vi "Keithley 648X Series Alternating Voltage Resistance Test.vi"() -> ()   [LabVIEW 2021]
doc: "This example shows how to configure a measurement, set up triggering, trigger a measurement, and retrieve a measurement. It shows how to use the low-level Data VIs to retrieve data from the instrument.\n\n<b>Note:</b>\nThis VI is only valid for Keithley 6487."
uses:
  <instrlib>/Keithley 648X Series/Keithley 648X Series.lvlib
panel:
  in  "Upper Measurement Range":u16(ring) items=["20mA", "2mA", "200uA", "20uA", "2uA", "200nA", "20nA", "2nA"]
  out "AV Measurement Results":cluster{dbl[], dbl[]}(graph)
  out "AV Amplitude Results":dbl[](array[numeric])
  in  "Enable Zero Check":bool
  in  "Measurement Time":dbl=6.0
  in  "Enable One Shot Mode":bool
  in  "AV Units":u16(ring)=1 items=["Amps", "Ohms"]
  in  "AV Measurement Cycles":i32=5
  in  "AV Pulse Time":dbl=10.0
  in  "AV High Voltage":dbl=5.0
  in  "Serial Configuration":T1={"Baud Rate"=9600, "Parity"=0, "Data Bits"=8, "Stop Bits"=10, "Flow Control"=0} {"Flow Control" items=["None", "XON/XOFF", "RTS/CTS", "XON/XOFF & RTS/CTS", "DTR/DSR", "XON/XOFF & DTR/DSR"]; "Stop Bits" items=["1.0"=10, "1.5"=15, "2.0"=20]; "Data Bits" items=["7"=7, "8"=8]; "Parity" items=["None", "Odd", "Even", "Mark", "Space"]; "Baud Rate" items=["300"=300, "600"=600, "1200"=1200, "2400"=2400, "4800"=4800, "9600"=9600, "19200"=19200]}
  in  "VISA resource name":refnum<visa-resource-name>
  # "(c) 2017 National Instruments.  ALL RIGHTS RESERVED."
  # "Measurement time is restricted\nto  0.02, 0.1, 1, 6, and 60 PLC\nduring A-V ohms mode."
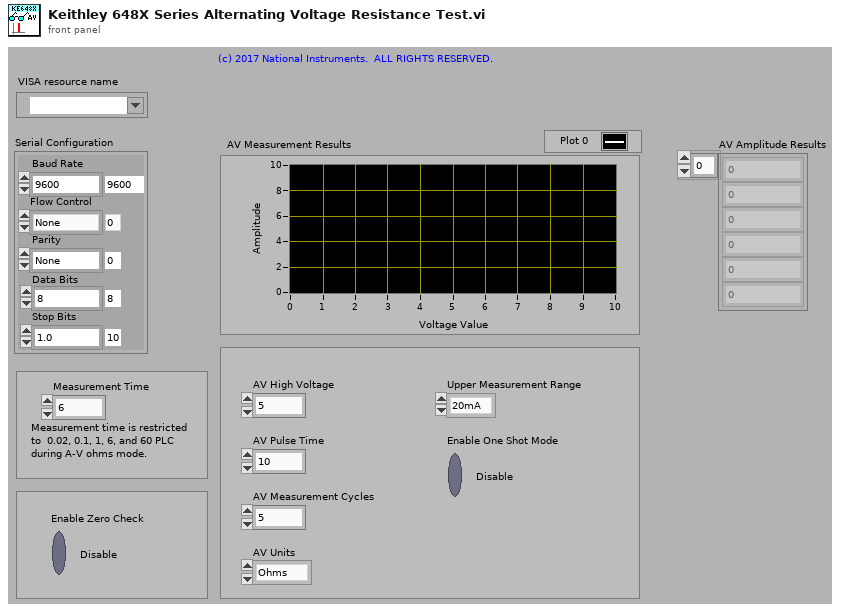
[diagram p1: front panel]
types:
  T1 = cluster{"Baud Rate":u32, "Parity":u16, "Data Bits":u16, "Stop Bits":u16, "Flow Control":u16}
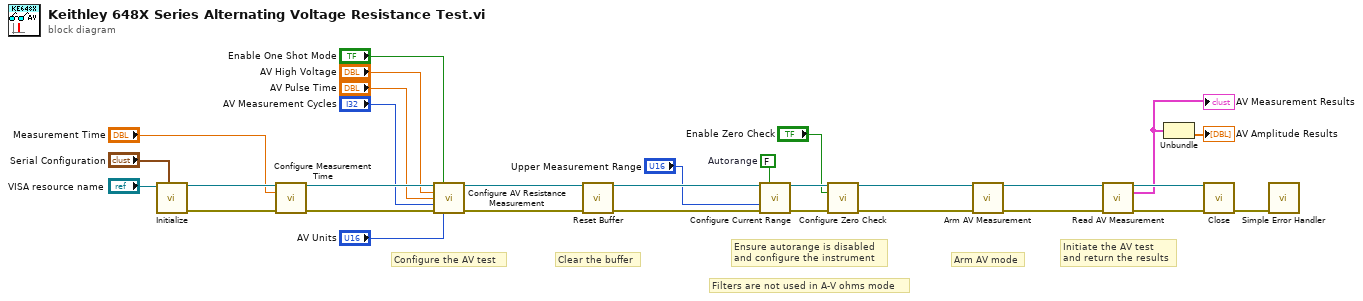
[diagram p0: block diagram]
diagram:
  w23 = FALSE  # Autorange
  # "Clear the buffer"
  # "Configure the AV test"
  # "Initiate the AV test\nand return the results"
  # "Arm AV mode"
  # "Ensure autorange is disabled\nand configure the instrument"
  # "Filters are not used in A-V ohms mode"
  n1 = call <instrlib>:"Initialize.vi"("Serial Configuration"="Serial Configuration", "VISA resource name"="VISA resource name") -> ("error out"=w12:errorcluster, "VISA resource name out"=w13:refnum<visa-resource-name>)  [unwired: 8 in]
  n2 = call <instrlib>:"Configure Measurement Time.vi"("VISA resource name"=w13, "Measurement Time (6 PLC)"="Measurement Time", "error in (no error)"=w12) -> ("VISA resource name out"=w10:refnum<visa-resource-name>, "error out"=w11:errorcluster)  [unwired: 11 in]
  n3 = call <instrlib>:"Configure AV Resistance Measurement.vi"("VISA resource name"=w10, "Enable One Shot Mode (T: Enable)"="Enable One Shot Mode", "AV High Voltage (10 V)"="AV High Voltage", "AV Pulse Time (1 s)"="AV Pulse Time", "AV Measurement Cycles (3)"="AV Measurement Cycles", "error in (no error)"=w11, "AV Units (0: Amps)"="AV Units") -> ("VISA resource name out"=w17:refnum<visa-resource-name>, "error out"=w18:errorcluster)  [unwired: 7 in]
  n4 = call <instrlib>:"Reset Buffer.vi"("VISA resource name"=w17, "error in (no error)"=w18) -> ("VISA resource name out"=w15:refnum<visa-resource-name>, "error out"=w16:errorcluster)  [unwired: 12 in]
  n5 = call <instrlib>:"Configure Current Range.vi"("VISA resource name"=w15, "Autorange (T: Enable)"=w23, "Upper Measurement Range (200uA)"="Upper Measurement Range", "error in (no error)"=w16) -> ("VISA resource name out"=w22:refnum<visa-resource-name>, "error out"=w21:errorcluster)  [unwired: 10 in]
  n6 = call <instrlib>:"Configure Zero Check.vi"("VISA resource name"=w22, "Enable Zero Check (T: Enable)"="Enable Zero Check", "error in (no error)"=w21) -> ("VISA resource name out"=w19:refnum<visa-resource-name>, "error out"=w20:errorcluster)  [unwired: 11 in]
  n7 = call <instrlib>:"Arm AV Measurement.vi"("VISA resource name"=w19, "error in (no error)"=w20) -> ("VISA resource name out"=w27:refnum<visa-resource-name>, "error out"=w24:errorcluster)  [unwired: 12 in]
  n8 = call <instrlib>:"Read AV Measurement.vi"("VISA resource name"=w27, "error in (no error)"=w24) -> ("VISA resource name out"=w26:refnum<visa-resource-name>, "AV Measurement Results"=w9:cluster{dbl[], dbl[]}, "error out"=w25:errorcluster)  [unwired: 11 in]
  "AV Measurement Results" <- w9
  n9 = Unbundle(w9) -> (→"AV Amplitude Results":dbl[])  [unwired: 1 out]
  n10 = call <instrlib>:"Close.vi"("error in (no error)"=w25, "VISA resource name"=w26) -> ("error out"=w29:errorcluster)  [unwired: 9 in]
  n11 = call <vilib>:"Simple Error Handler.vi"("error in (no error)"=w29) -> ()  [unwired: 4 in, 5 out]
